vi "m1m3_logEvent_AppliedStaticForces.vi"(8 "error in (no error)":errorcluster, 11 "logevent_AppliedStaticForces_Ctl":T1) -> (0 "error out":errorcluster, 2 "function return":i32, 3 "logevent_AppliedStaticForces_Ctl out":T1)   [LabVIEW 2016, in "SALLV_m1m3.lvlib"]
doc: "int m1m3_shm_logEvent_AppliedStaticForcesLV(m1m3_logevent_AppliedStaticForcesLV *logevent_AppliedStaticForces_Ctl );"
uses:
  SALLV_m1m3.lvlib
  DataTypes/logevent_AppliedStaticForces.ctl
  SALLV_m1m3.so
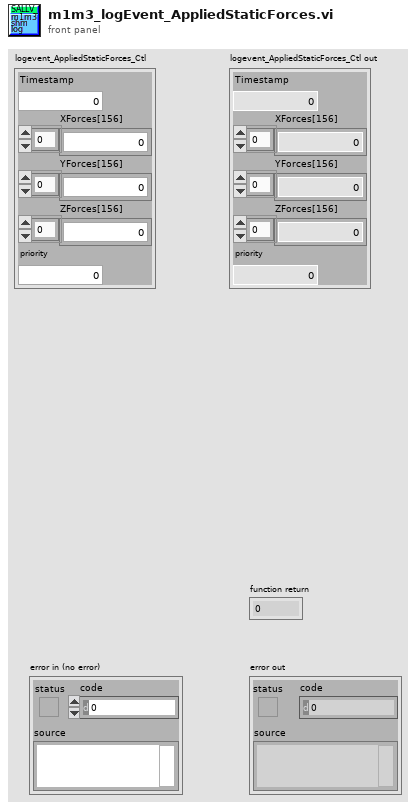
[diagram p1: front panel]
types:
  T1 = typedef "SALLV_m1m3.lvlib/logevent_AppliedStaticForces.ctl" = cluster{"Timestamp":dbl, "XForces[156]":dbl[], "YForces[156]":dbl[], "ZForces[156]":dbl[], "priority":i32}
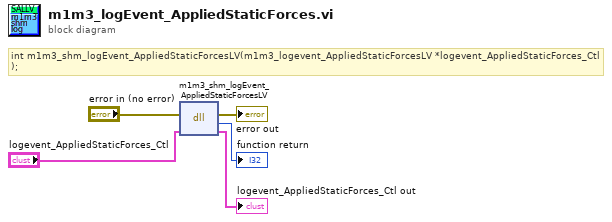
[diagram p0: block diagram]
diagram:
  # "int m1m3_shm_logEvent_AppliedStaticForcesLV(m1m3_logevent_AppliedStaticForcesLV *logevent_AppliedStaticForces_Ctl );"
  n1 = dll-call lib="opt/CODE/SALLV_m1m3/SALLV_m1m3.*" fn="m1m3_shm_logEvent_AppliedStaticForcesLV"(error in="error in (no error)", "logevent_AppliedStaticForces_Ctl"="logevent_AppliedStaticForces_Ctl") -> (error out=→"error out":errorcluster, →"function return":i32, "logevent_AppliedStaticForces_Ctl"=→"logevent_AppliedStaticForces_Ctl out":T1)  [unwired: 2 in, 1 out]
